vi "Sample Transfer Reset to Idle.vi"(6 "Echo (True)":bool=TRUE, 8 "error in (no error)":errorcluster, 11 "cRIO-CO2 in":refnum<class "cRIO-CO2.lvclass">) -> (0 "error out":errorcluster, 3 "cRIO-CO2 out":refnum<class "cRIO-CO2.lvclass">)   [LabVIEW 2015, in "cRIO-Carbondioxide.lvlib" / "cRIO-CO2.lvlib" / "cRIO-CO2.lvclass"]
uses:
  cRIO-CO2.lvclass
  <vilib>/ActorFramework/Time-Delayed Send Message/Time-Delay Override Options.ctl
  Controls/Sample Transfer State Enumerator.ctl
  Controls/Sample Transfer Container Enumerator.ctl
  subs/Sample/Sample.lvclass
  cRIO-CO2.lvclass/cRIO-CO2.ctl
  Send Time-delayed Transfer Sample.vi
  State Elapsed Time.vi
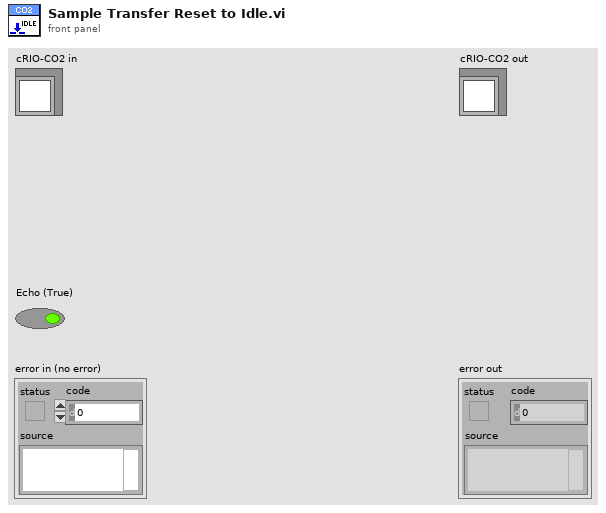
[diagram p1: front panel]
types:
  T1 = typedef "Sample Transfer State Enumerator.ctl" = enum16{"Idle", "Initialize", "Check Containers", "Check Temperatures", "Start Turbo", "Warm Up Containers", "Prepare for purging", "Purge Capillary", "Purge", "Open Containers", "Introduce Sample", "Measure Base Pressure", "Home Syringe", "Start Freezer", "Freeze Target", "Crystalize", "Initiate Stash", "Stash", "Polish", "Stop Freezers", "Push Sample", "Complete", "Abort", "Error", "Undefined"}
  T2 = typedef "Time-Delay Override Options.ctl" = enum16{"Send next copy now", "Skip next scheduled copy", "Send next copy now and stop all further copies", "Stop all further copies"}
  T3 = typedef "Sample Transfer Container Enumerator.ctl" = enum16{"None", "Sample 1", "Sample 2", "Sample 3", "Sample 4", "Sample 5", "Storage 01", "Storage 02", "Storage 03", "Storage 04", "Storage 05", "Storage 06", "Storage 07", "Storage 08", "Storage 09", "Storage 10", "Storage 11", "Storage 12", "Syringe", "Undefined"}
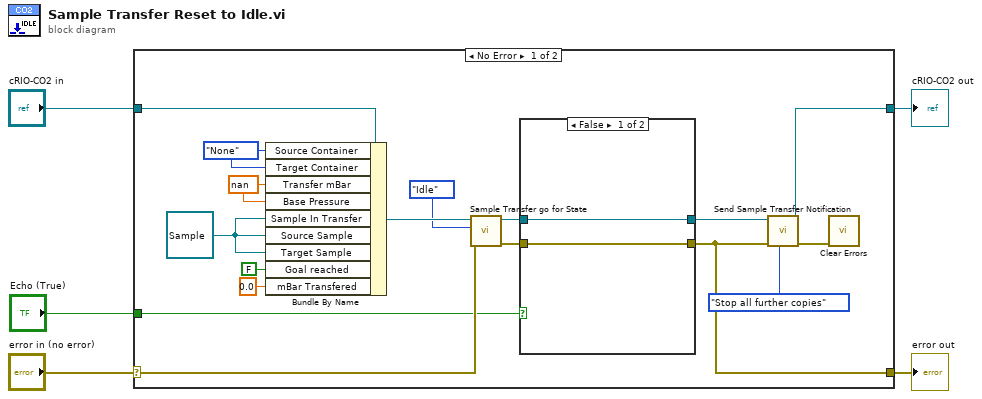
[diagram p0: block diagram]
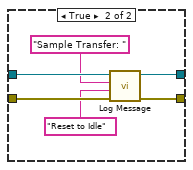
[diagram p2: hidden frame]
diagram:
  n1 = case shown="No Error" "error in (no error)" {
    selector: "error in (no error)" -> [w22 w32]
    tunnel: [w7 w32] -> w4
    tunnel: [w19 w31] -> w2
    tunnel: "cRIO-CO2 in" -> [w10 w31]
    tunnel: "Echo (True)" -> [w6 _]
    frame No Error {
      w13 = refnum<class "Sample.lvclass"> refnum ("Sample Transfer.Samples.Sample In Transfer")
      w14 = nan ("Sample Transfer.Transfer mBar")
      w15 = Sample_Transfer_Container_Enumerator."None" ("Sample Transfer.Source Container")
      n2 = Bundle By Name(cluster=w10, "Source Container"=w15, "Target Container"=w15, "Transfer mBar"=w14, "Base Pressure"=w14, "Sample In Transfer"=w13, "Source Sample"=w13, "Target Sample"=w13, "Goal reached"=FALSE ("Sample Transfer.Goal reached"), "mBar Transfered"=0.0 ("Sample Transfer.mBar Transfered")) -> (w9:refnum<class "cRIO-CO2.lvclass">)
      n3 = call "Sample Transfer go for State.vi"("error in (no error)"=w22, "Sample Transfer State"=Sample_Transfer_State_Enumerator."Idle", "cRIO-CO2 in"=w9) -> ("error out"=w18:errorcluster, "cRIO-CO2 out"=w17:refnum<class "cRIO-CO2.lvclass">)  [unwired: 7 in]
      n4 = case shown="False" w6 {
        tunnel: w18 -> [w23 w30]
        tunnel: w17 -> [w24 w29]
        tunnel: [w24 w26] -> w16
        tunnel: [w23 w25] -> w7
        frame False {
        }
        frame True {
          n5 = call "Log Message.vi"("error in (no error)"=w30, "String"="Reset to Idle", "Source Name"="Sample Transfer: ", "cRIO-CO2 in"=w29) -> ("error out"=w25:errorcluster, "cRIO-CO2 out"=w26:refnum<class "cRIO-CO2.lvclass">)  [unwired: 6 in]
        }
      }
      n6 = call "Send Sample Transfer Notification.vi"("notification (Send next copy now)"=Time-Delay_Override_Options."Stop all further copies", "error in (no error)"=w7, "cRIO-CO2 in"=w16) -> ("error out"=w21:errorcluster, "cRIO-CO2 out"=w19:refnum<class "cRIO-CO2.lvclass">)  [unwired: 7 in]
      n7 = call <vilib>:"Clear Errors.vi"("error in (no error)"=w21) -> ()  [unwired: 5 in, 2 out]
    }
    frame Error {
    }
  }
  "error out" <- w4
  "cRIO-CO2 out" <- w2
